vi "genArmDisarmPacket.vi"(10 "node ID":u8, 11 "state":bool) -> (3 "packet string":string)   [LabVIEW 2011]
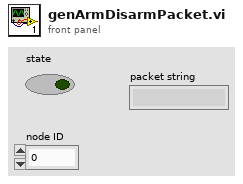
[diagram p1: front panel]
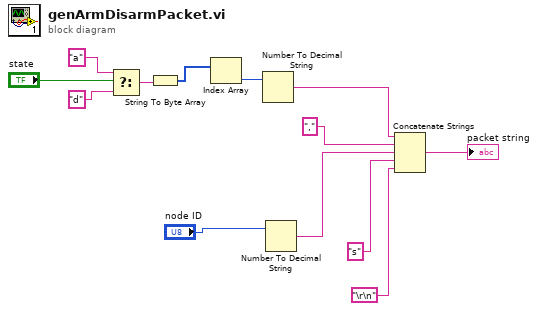
[diagram p0: block diagram]
diagram:
  n1 = Select(t="a", s="state", f="d") -> (s? t:f=w7:string)
  n2 = String To Byte Array(string=w7) -> (unsigned byte array=w13:u8[])
  n3 = Index Array(array=w13) -> (element=w12:u8)  [unwired: 1 in]
  n4 = Number To Decimal String(number=w12) -> (decimal integer string=w10:string)  [unwired: 1 in]
  n5 = Number To Decimal String(number="node ID") -> (decimal integer string=w3:string)  [unwired: 1 in]
  n6 = Concatenate Strings(w10, ",", w3, "s", "\r\n") -> (→"packet string":string)
